vi "Update TC Temperature.vi"(8 "error in":errorcluster, 10 "TC Temperature":waveform(dbl)[](array[waveform]), 11 "DeepU Results in":refnum<class "DeepU Results.lvclass">) -> (0 "error out":errorcluster, 3 "DeepU Results out":refnum<class "DeepU Results.lvclass">)   [LabVIEW 2019, in "Results.lvlib" / "DeepU Results.lvclass"]
uses:
  DeepU Results.lvclass
  DeepU Results.lvclass/DeepU Results.ctl
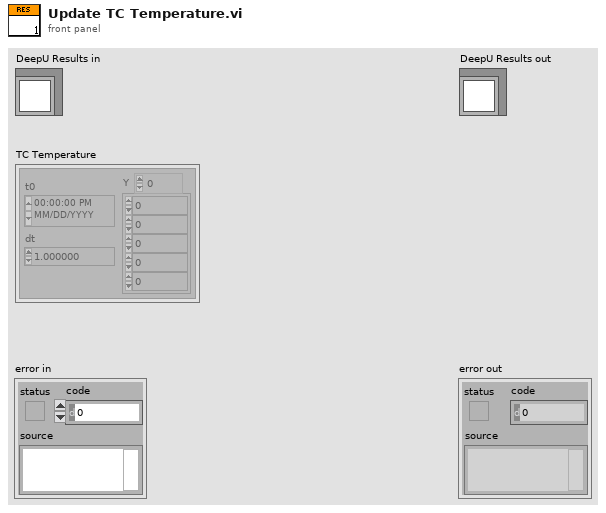
[diagram p1: front panel]
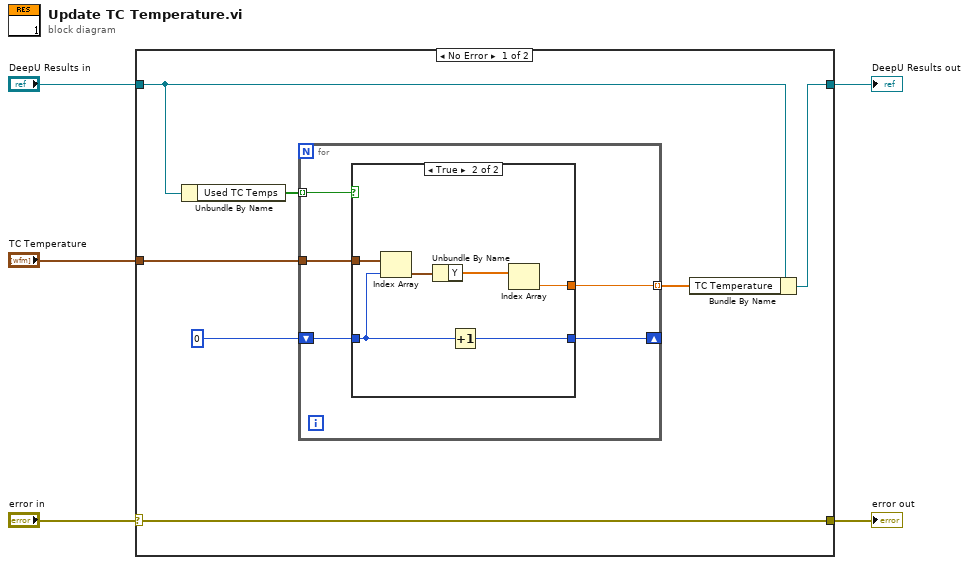
[diagram p0: block diagram]
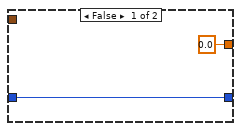
[diagram p2: hidden frame]
diagram:
  n1 = case shown="No Error" "error in" {
    selector: "error in" -> [w12 w26]
    tunnel: [w12 w26] -> w1
    tunnel: [w11 w27] -> w2
    tunnel: "DeepU Results in" -> [w10 w27]
    tunnel: "TC Temperature" -> [w9 _]
    frame No Error {
      n2 = Unbundle By Name(w10) -> ("Used TC Temps"=w7:bool[])
      n3 = for {
        tunnel: w7 -> [w16] mode=indexing
        tunnel: w9 -> [w17]
        shift-right: [w14] -> _
        shift-left: 0 -> [w15]
        tunnel: [w13] -> w6 mode=indexing
        n4 = case shown="True" w16 {
          tunnel: w17 -> [_ w25]
          tunnel: w15 -> [w19 w24]
          tunnel: [w19 w23] -> w14
          tunnel: [0.0 w20] -> w13
          frame False {
          }
          frame True {
            n5 = Index Array(array=w25, index=w24) -> (element=w22:waveform(dbl))
            n6 = Unbundle By Name(w22) -> ("Y"=w21:dbl[])
            n7 = Increment(x=w24) -> (x+1=w23:i32)
            n8 = Index Array(array=w21) -> (element=w20:dbl)  [unwired: 1 in]
          }
        }
      }
      n9 = Bundle By Name(cluster=w10, "TC Temperature"=w6) -> (w11:refnum<class "DeepU Results.lvclass">)
    }
    frame Error {
    }
  }
  "error out" <- w1
  "DeepU Results out" <- w2
